vi "PTSequencer.start.vi"(0 "i ref in":refnum<vi>, 3 "ms timeout (10000)":i32=10000, 5 "error in (no error)":errorcluster) -> (14 "i ref out":refnum<vi>, 16 "next step":string, 17 "timed out":bool, 19 "error out":errorcluster)   [LabVIEW 2014, in "PTSequencer.lvlib"]
uses:
  PTSequencer.lvlib
  CS_Core/BaseSM/BaseSM.lvlib
  CSlibraries-extern/DimLVEvent/LVDimInterface/LVDimInterface.lvlib
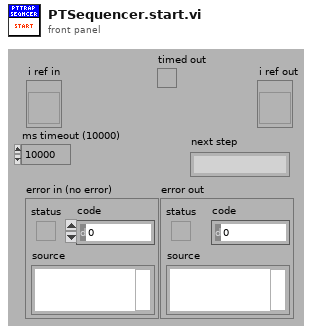
[diagram p1: front panel]
types:
  T1 = typedef "PTSequencer.lvlib/PTSequencer.i attribute.ctl" = cluster{"subsequence":bool, "mode":T2, "i step":i32, "nofLoops":i32, "i loop":i32, "Running":bool, "Paused":bool, "step done":bool, "loop done":bool, "seq done":bool, "DIM IDs":cluster{"step done":i32, "loop done":i32, "seq done":i32, "i step":i32, "i loop":i32}, "use stop conditions":bool, "stop conditions":T3[], "Step List":T5[], "DIM subsriptions":string[], "stop cond indexes":i32[], "step cond indexes":cluster{"step condition IDs":cluster{"step ID":i32, "condition ID":i32}[]}[], "Delay Start Time":timestamp, "status":string, "stopping":bool}
  T2 = typedef "PTSequencer.lvlib/PTSequencer.mode.ctl" = enum16{"single", "loop", "for loop"}
  T3 = typedef "PTSequencer.lvlib/PTSequencer.DIM service condition.ctl" = cluster{"DIM service":string, "descr":string, "nomValue":T4, "actValue":T4, "matched":bool, "DIM Status":cluster{"no link":bool, "quality":i32, "Time Stamp":timestamp}}
  T4 = typedef "CoreDefs.rawDataType.ctl" = i8[]
  T5 = typedef "PTSequencer.lvlib/PTSequencer.step.ctl" = cluster{"description":string, "object parameters":cluster{"object":string, "selector":string, "descriptor":string, "data":T4, "subsequence":bool, "call mode":enum16{"Simple DIM", "Synchronous"}, "data in":T4}, "result action":cluster{"check":bool, "passed":enum16{"Next", "Previous", "Repeat", "Jump"}, "failed":enum16{"Next", "Previous", "Repeat", "Jump"}, "jumpID_passed":i32, "jumpID_failed":i32}, "conditions":T3[], "fulfilled ":bool, "use delay":bool, "delay time (s)":dbl, "ID":i32}
  T6 = cluster{"step done":i32, "loop done":i32, "seq done":i32, "i step":i32, "i loop":i32}
  T7 = typedef "BaseSM.lvlib/BaseSM.i attribute.ctl" = cluster{"stateError":i32, "stateStatus":string, "stateQuality":T8, "ProcStateRef":refnum<vi>, "thread ref":refnum<vi>, "actState":string, "reqState":string, "SMQueue":refnum<queue>, "stateErrorID":i32, "stateStatusID":i32}
  T8 = typedef "BaseSM.lvlib/BaseSM.stateQuality.ctl" = i16
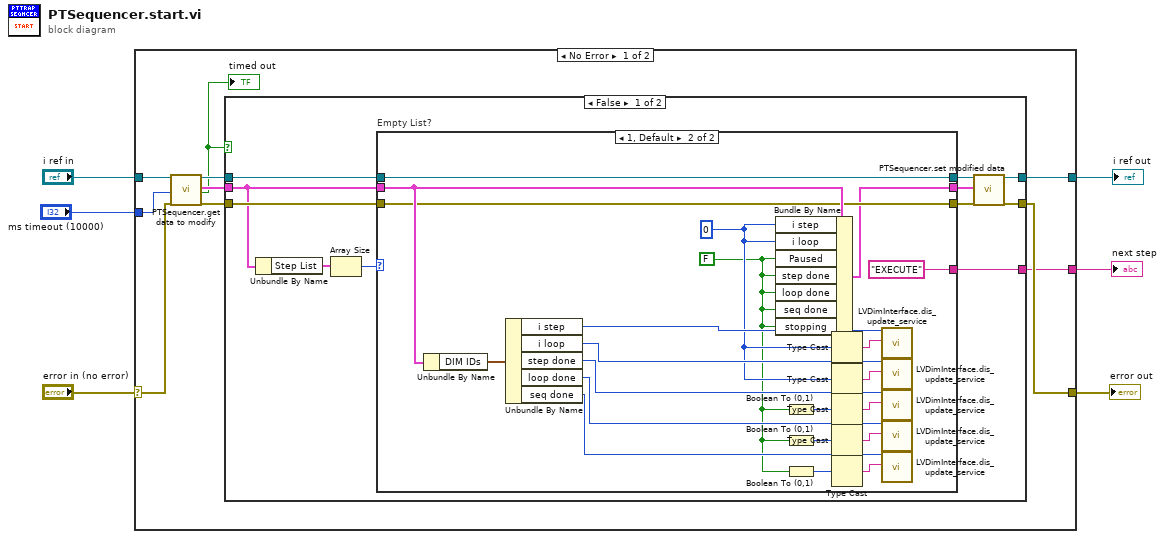
[diagram p0: block diagram]
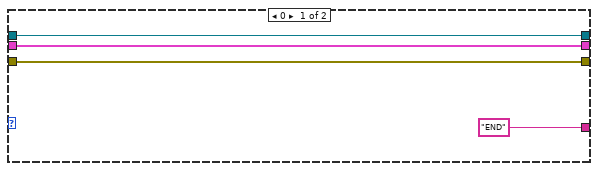
[diagram p2: hidden frame]
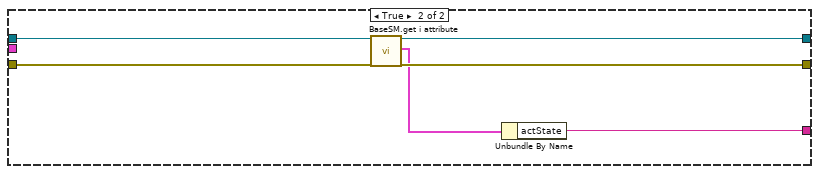
[diagram p3: hidden frame]
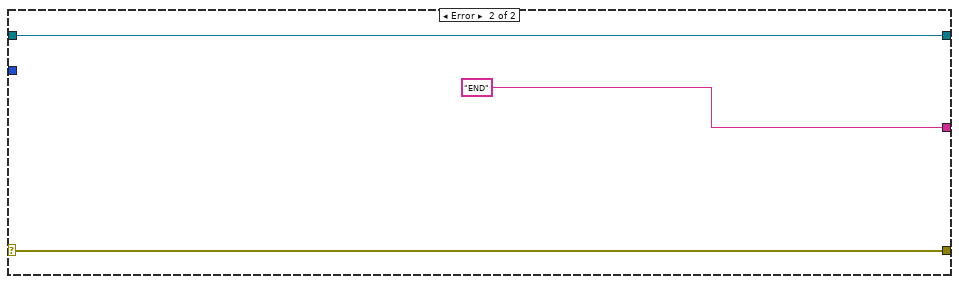
[diagram p4: hidden frame]
diagram:
  n1 = case shown="No Error" "error in (no error)" {
    selector: "error in (no error)" -> [w12 w60]
    tunnel: "i ref in" -> [w16 w61]
    tunnel: [w10 w60] -> w5
    tunnel: [w11 w61] -> w4
    tunnel: "ms timeout (10000)" -> [w8 _]
    tunnel: [w7 "END"] -> w1
    frame No Error {
      n2 = call "PTSequencer.get data to modify.vi"("i ref in"=w16, "ms timeout (10000)"=w8, "error in (no error)"=w12) -> ("i ref out"=w13:refnum<vi>, "i attribute"=w15:T1, "timed out"=w9:bool, "error out"=w14:errorcluster)  [unwired: 13 in]
      "timed out" <- w9
      n3 = case shown="False" w9 {
        tunnel: w15 -> [w21 _]
        tunnel: w14 -> [w22 w56]
        tunnel: w13 -> [w23 w58]
        tunnel: [w27 w55] -> w11
        tunnel: [w26 w57] -> w10
        tunnel: [w18 w53] -> w7
        frame False {
          n4 = Unbundle By Name(w21) -> ("Step List"=w25:T5[])
          n5 = Array Size(array=w25) -> (size(s)=w24:i32)
          n6 = case "Empty List?" shown="1, Default" w24 {
            tunnel: w23 -> [w31 w39]
            tunnel: w22 -> [w30 w40]
            tunnel: w21 -> [w28 w52]
            tunnel: [w30 w40] -> w20
            tunnel: [w31 w39] -> w19
            tunnel: ["END" "EXECUTE"] -> w18
            tunnel: [w28 w38] -> w17
            frame 0 {
            }
            frame 1, Default {
              w32 = FALSE ("Paused")
              w33 = 0 ("i step")
              n7 = Unbundle By Name(w52) -> ("DIM IDs"=w51:T6)
              n8 = Unbundle By Name(w51) -> ("i step"=w50:i32, "i loop"=w49:i32, "step done"=w48:i32, "loop done"=w47:i32, "seq done"=w46:i32)
              n9 = Bundle By Name(cluster=w52, "i step"=w33, "i loop"=w33, "Paused"=w32, "step done"=w32, "loop done"=w32, "seq done"=w32, "stopping"=w32) -> (w38:T1)
              n10 = Boolean To (0,1)(Boolean=w32) -> (0, 1=w35:i16)
              n11 = Boolean To (0,1)(Boolean=w32) -> (0, 1=w36:i16)
              n12 = Boolean To (0,1)(Boolean=w32) -> (0, 1=w37:i16)
              n13 = Type Cast(x=w33) -> (*(type *) &x=w45:string)  [unwired: 1 in]
              n14 = Type Cast(x=w33) -> (*(type *) &x=w44:string)  [unwired: 1 in]
              n15 = Type Cast(x=w35) -> (*(type *) &x=w43:string)  [unwired: 1 in]
              n16 = Type Cast(x=w36) -> (*(type *) &x=w42:string)  [unwired: 1 in]
              n17 = Type Cast(x=w37) -> (*(type *) &x=w41:string)  [unwired: 1 in]
              n18 = call "LVDimInterface.dis_update_service.vi"("my_serviceID"=w50, "data"=w45) -> ()  [unwired: 15 in, 3 out]
              n19 = call "LVDimInterface.dis_update_service.vi"("my_serviceID"=w49, "data"=w44) -> ()  [unwired: 15 in, 3 out]
              n20 = call "LVDimInterface.dis_update_service.vi"("my_serviceID"=w48, "data"=w43) -> ()  [unwired: 15 in, 3 out]
              n21 = call "LVDimInterface.dis_update_service.vi"("my_serviceID"=w47, "data"=w42) -> ()  [unwired: 15 in, 3 out]
              n22 = call "LVDimInterface.dis_update_service.vi"("my_serviceID"=w46, "data"=w41) -> ()  [unwired: 15 in, 3 out]
            }
          }
          n23 = call "PTSequencer.set modified data.vi"("i ref in"=w19, "CLASS.i attribute"=w17, "error in (no error)"=w20) -> ("i ref out"=w27:refnum<vi>, "error out"=w26:errorcluster)  [unwired: 15 in]
        }
        frame True {
          n24 = call "BaseSM.get i attribute.vi"("i ref in"=w58, "error in (no error)"=w56) -> ("i ref out"=w55:refnum<vi>, "i attribute"=w54:T7, "error out"=w57:errorcluster)  [unwired: 15 in]
          n25 = Unbundle By Name(w54) -> ("actState"=w53:string)
        }
      }
    }
    frame Error {
    }
  }
  "error out" <- w5
  "i ref out" <- w4
  "next step" <- w1
